vi "Periodic Tasks.vi"(11 "error in (no error)":errorcluster) -> ()   [LabVIEW 2012]
doc: "This VI runs in parallel to other tasks. It can contain as many user-defined periodic loops as you need. These can carry out PID or other sorts of timed response."
uses:
  <vilib>/Rock Robotics/WPI/DriverStation/DriverStationLCD/WPI_DriverStationLCDLCDLine.ctl
  <vilib>/Rock Robotics/SystemInterfaces/Utilities/FPGA_UtilitiesLED Source.ctl
  <vilib>/Rock Robotics/SystemInterfaces/Utilities/FPGA_UtilitiesLED State.ctl
  Robot Global Data.vi
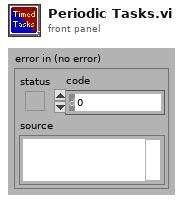
[diagram p1: front panel]
types:
  T1 = typedef "WPI_DriverStationLCDLCDLine.ctl" = enum16{"Main - Line 1", "User - Line 2", "User - Line 3", "User - Line 4", "User - Line 5", "User - Line 6"}
  T2 = cluster{"Case":dbl, "VisionTrack":bool, "ShootEnableWheels":bool, "Shoot":bool, "ManualExtend":dbl, "ManualRotate":dbl, "YCoord":dbl, "FlipUp":bool, "RotDeadband":dbl, "ExtDeadband":dbl, "ExtPOT":dbl, "RotPOT":dbl, "WheelFSpd":dbl, "WheelBSpd":dbl, "ServoPositions":cluster{"FlipperLeftUp":dbl, "FlipperLeftDown":dbl, "FlipperRightUp":dbl, "FlipperRightDown":dbl, "KickerLeftBack":dbl, "KickerLeftForward":dbl, "KickerRightBack":dbl, "KickerRightForward":dbl}, "POTPositions":cluster{"Setpoint 1":dbl, "Setpoint 2":dbl, "Setpoint 3":dbl, "Setpoint 4":dbl, "RotLow":dbl, "RotHigh":dbl, "ExtLow":dbl, "ExtHigh":dbl}, "ClimberHooked":bool}
  T3 = typedef "WPI_DigitalInputDevRef.ctl" = cluster{"DevStatus":errorcluster, "DIO Channel":T4, "Digital Module":T5}
  T4 = typedef "FPGA_DIOChannel.ctl" = enum8{"DIO 1", "DIO 2", "DIO 3", "DIO 4", "DIO 5", "DIO 6", "DIO 7", "DIO 8", "DIO 9", "DIO 10", "DIO 11", "DIO 12", "DIO 13", "DIO 14", "Invalid"}
  T5 = typedef "FPGA_TypedefDigitalModule.ctl" = enum16{"Digital Module 1", "Digital Module 2"}
  T6 = typedef "WPI_AnalogChannelDevRef.ctl" = cluster{"DevStatus":errorcluster, "Analog Module":T7, "Analog Channel":T8}
  T7 = typedef "FPGA_TypedefAnalogModule.ctl" = enum16{"Analog Module 1", "Analog Module 2"}
  T8 = typedef "FPGA_AIChannel.ctl" = enum8{"AI 1", "AI 2", "AI 3", "AI 4", "AI 5", "AI 6", "AI 7", "AI 8", "Invalid"}
  T9 = cluster{"FlipperLeftUp":dbl, "FlipperLeftDown":dbl, "FlipperRightUp":dbl, "FlipperRightDown":dbl, "KickerLeftBack":dbl, "KickerLeftForward":dbl, "KickerRightBack":dbl, "KickerRightForward":dbl}
  T10 = cluster{"Setpoint 1":dbl, "Setpoint 2":dbl, "Setpoint 3":dbl, "Setpoint 4":dbl, "RotLow":dbl, "RotHigh":dbl, "ExtLow":dbl, "ExtHigh":dbl}
  T11 = typedef "WPI_GyroDevRef.ctl" = cluster{"DevStatus":errorcluster, "Analog Module":T7, "Analog Channel":T8, "Offset":dbl, "Gain (VoltsPerDegree/Second)":dbl}
  T12 = typedef "WPI_EncoderDevRef.ctl" = cluster{"DevStatus":errorcluster, "EncoderIndex":T13, "CounterIndex":T14, "DistancePerCount":dbl, "Decoding Type":T15}
  T13 = typedef "FPGA_EncoderIdx.ctl" = enum8{"Enc 0", "Enc 1", "Enc 2", "Enc 3", "Invalid"}
  T14 = typedef "FPGA_CounterCtrSystemIndex.ctl" = enum8{"Ctr 0", "Ctr 1", "Ctr 2", "Ctr 3", "Ctr 4", "Ctr 5", "Ctr 6", "Ctr 7", "Invalid"}
  T15 = typedef "WPI_EncoderType.ctl" = enum16{"1x", "2x", "4x"}
  T16 = typedef "WPI_RelayValue.ctl" = enum16{"Off", "On", "Forward", "Reverse"}
  T17 = cluster{"Case":dbl, "Extension":dbl, "Rotation":dbl, "WheelF":dbl, "WheelB":dbl, "Left Kicker":dbl, "Right Kicker":dbl, "Left Flipper":dbl, "Right Flipper":dbl, "Lights":T16}
  T18 = typedef "FPGA_UtilitiesLED State.ctl" = enum16{"Off", "On", "Toggle"}
  T19 = typedef "FPGA_UtilitiesLED Source.ctl" = enum16{"User LED", "FPGA LED"}
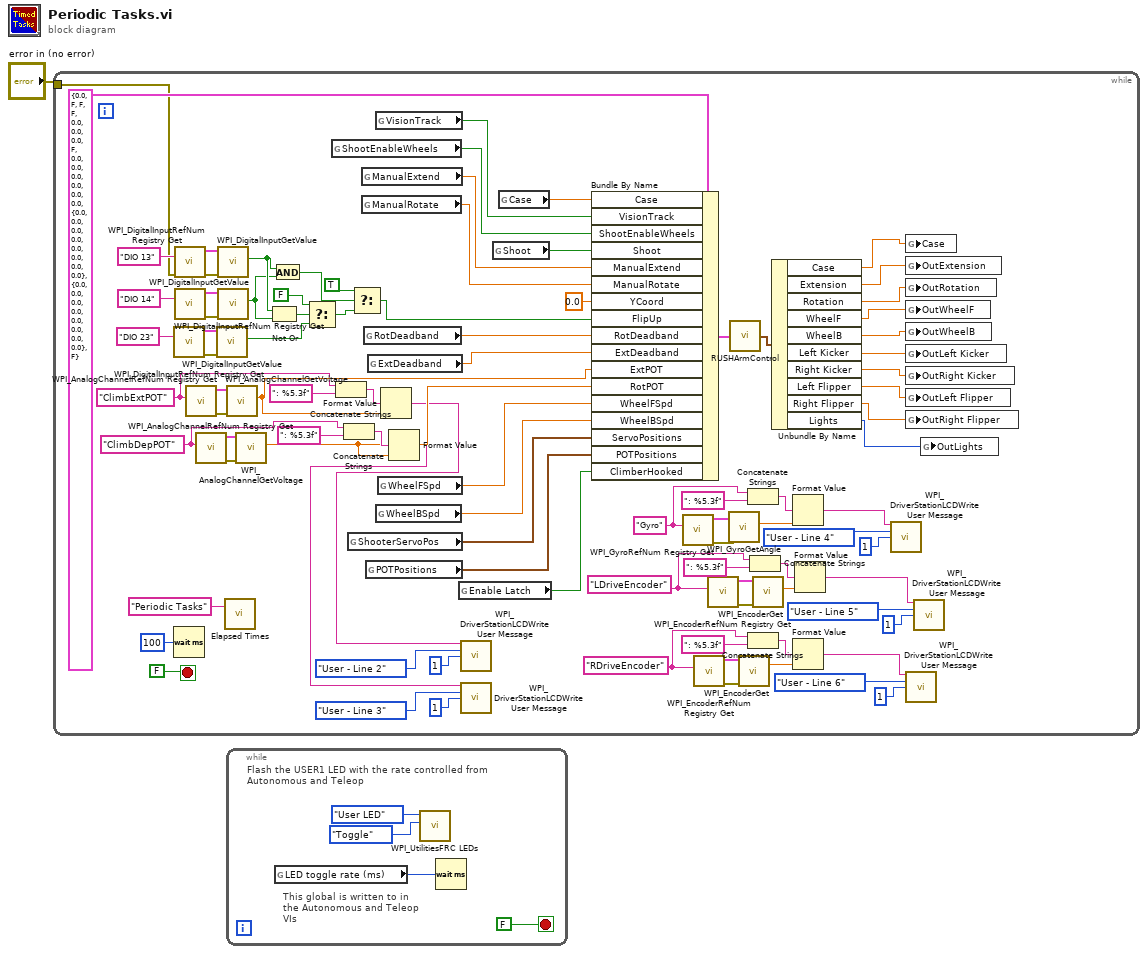
[diagram p0: block diagram]
diagram:
  n1 = while {
    tunnel: "error in (no error)" -> [w38]
    stop <- FALSE stop-if-true
    w8 = "ClimbExtPOT" ("refnum name")
    w19 = "RDriveEncoder" ("refnum name")
    w13 = "LDriveEncoder" ("refnum name")
    w4 = "ClimbDepPOT" ("refnum name")
    w31 = "Gyro" ("refnum name")
    n2 = call <vilib>:"WPI_DigitalInputRefNum Registry Get.vi"("refnum name"="DIO 23") -> ("error out"=w44:errorcluster, "DigitalInputDevRef"=w41:T3)  [unwired: 9 in]
    n3 = Wait (ms)(milliseconds to wait=u32 100) -> ()  [unwired: 1 out]
    n4 = call <vilib>:"WPI_DigitalInputRefNum Registry Get.vi"("error in (no error)"=w38, "refnum name"="DIO 13") -> ("error out"=w58:errorcluster, "DigitalInputDevRef"=w57:T3)  [unwired: 8 in]
    n5 = call <vilib>:"WPI_DigitalInputRefNum Registry Get.vi"("refnum name"="DIO 14") -> ("error out"=w53:errorcluster, "DigitalInputDevRef"=w54:T3)  [unwired: 9 in]
    n6 = call <vilib>:"WPI_AnalogChannelRefNum Registry Get.vi"("refnum name"=w8) -> ("error out"=w90:errorcluster, "AIDeviceRef"=w39:T6)  [unwired: 9 in]
    n7 = call <vilib>:"WPI_AnalogChannelRefNum Registry Get.vi"("refnum name"=w4) -> ("error out"=w85:errorcluster, "AIDeviceRef"=w84:T6)  [unwired: 9 in]
    n8 = call <vilib>:"WPI_DigitalInputGetValue.vi"("error in (no error)"=w44, "DigitalInputDevRef"=w41) -> ("Value"=w42:bool)  [unwired: 7 in, 2 out]
    n9 = call <vilib>:"WPI_DigitalInputGetValue.vi"("error in (no error)"=w58, "DigitalInputDevRef"=w57) -> ("Value"=w50:bool)  [unwired: 7 in, 2 out]
    n10 = call <vilib>:"WPI_DigitalInputGetValue.vi"("error in (no error)"=w53, "DigitalInputDevRef"=w54) -> ("Value"=w49:bool)  [unwired: 7 in, 2 out]
    n11 = call "Elapsed Times.vi"("Call Name"="Periodic Tasks") -> ()  [unwired: 2 in, 1 out]
    n12 = call <vilib>:"WPI_AnalogChannelGetVoltage.vi"("error in (no error)"=w90, "AIDeviceRef"=w39) -> ("Voltage"=w9:dbl)  [unwired: 7 in, 2 out]
    n13 = call <vilib>:"WPI_AnalogChannelGetVoltage.vi"("error in (no error)"=w85, "AIDeviceRef"=w84) -> ("Voltage"=w5:dbl)  [unwired: 7 in, 2 out]
    n14 = Not Or(1:w49, 2:w50) -> (0:w48:bool)
    n15 = And(x=w50, y=w49) -> (x .and. y?=w52:bool)
    n16 = Select(t=FALSE, s=w48, f=w42) -> (s? t:f=w46:bool)
    n17 = global read "Robot Global Data.vi" "ShootEnableWheels"() -> (w78:bool)
    n18 = Concatenate Strings(w8, ": %5.3f") -> (w10:string)
    n19 = Concatenate Strings(w4, ": %5.3f") -> (w7:string)
    n20 = global read "Robot Global Data.vi" "ShooterServoPos"() -> (w70:T9)
    n21 = Select(t=TRUE, s=w52, f=w46) -> (s? t:f=w45:bool)
    n22 = global read "Robot Global Data.vi" "ManualExtend"() -> (w76:dbl)
    n23 = global read "Robot Global Data.vi" "ManualRotate"() -> (w75:dbl)
    n24 = global read "Robot Global Data.vi" "RotDeadband"() -> (w74:dbl)
    n25 = global read "Robot Global Data.vi" "POTPositions"() -> (w69:T10)
    n26 = global read "Robot Global Data.vi" "ExtDeadband"() -> (w73:dbl)
    n27 = global read "Robot Global Data.vi" "VisionTrack"() -> (w79:bool)
    n28 = global read "Robot Global Data.vi" "WheelBSpd"() -> (w71:dbl)
    n29 = global read "Robot Global Data.vi" "WheelFSpd"() -> (w72:dbl)
    n30 = Format Value(format string=w10, value (0)=w9) -> (output string=w3:string)  [unwired: 1 in]
    n31 = Format Value(format string=w7, value (0)=w5) -> (output string=w2:string)  [unwired: 1 in]
    n32 = global read "Robot Global Data.vi" "Enable Latch"() -> (w40:bool)
    n33 = call <vilib>:"WPI_DriverStationLCDWrite User Message.vi"("line text"=w3, "line"=WPI_DriverStationLCDLCDLine."User - Line 2", "starting column"=i8 1) -> ()  [unwired: 2 in, 11 out]
    n34 = call <vilib>:"WPI_DriverStationLCDWrite User Message.vi"("line text"=w2, "line"=WPI_DriverStationLCDLCDLine."User - Line 3", "starting column"=i8 1) -> ()  [unwired: 2 in, 11 out]
    n35 = global read "Robot Global Data.vi" "Shoot"() -> (w77:bool)
    n36 = global read "Robot Global Data.vi" "Case"() -> (w80:dbl)
    n37 = Bundle By Name(cluster=T2 {"Case"=0.0, "VisionTrack"=FALSE, "ShootEnableWheels"=FALSE, "Shoot"=FALSE, "ManualExtend"=0.0, "ManualRotate"=0.0, "YCoord"=0.0, "FlipUp"=FALSE, "RotDeadband"=0.0, "ExtDeadband"=0.0, "ExtPOT"=0.0, "RotPOT"=0.0, "WheelFSpd"=0.0, "WheelBSpd"=0.0, "ServoPositions"={"FlipperLeftUp"=0.0, "FlipperLeftDown"=0.0, "FlipperRightUp"=0.0, "FlipperRightDown"=0.0, "KickerLeftBack"=0.0, "KickerLeftForward"=0.0, "KickerRightBack"=0.0, "KickerRightForward"=0.0}, "POTPositions"={"Setpoint 1"=0.0, "Setpoint 2"=0.0, "Setpoint 3"=0.0, "Setpoint 4"=0.0, "RotLow"=0.0, "RotHigh"=0.0, "ExtLow"=0.0, "ExtHigh"=0.0}, "ClimberHooked"=FALSE} ("In Cluster"), "Case"=w80, "VisionTrack"=w79, "ShootEnableWheels"=w78, "Shoot"=w77, "ManualExtend"=w76, "ManualRotate"=w75, "YCoord"=0.0, "FlipUp"=w45, "RotDeadband"=w74, "ExtDeadband"=w73, "ExtPOT"=w9, "RotPOT"=w5, "WheelFSpd"=w72, "WheelBSpd"=w71, "ServoPositions"=w70, "POTPositions"=w69, "ClimberHooked"=w40) -> (w82:T2)
    n38 = call <vilib>:"WPI_GyroRefNum Registry Get.vi"("refnum name"=w31) -> ("error out"=w91:errorcluster, "GyroDevRef"=w92:T11)  [unwired: 9 in]
    n39 = call <vilib>:"WPI_EncoderRefNum Registry Get.vi"("refnum name"=w19) -> ("error out"=w87:errorcluster, "EncoderDevRef"=w86:T12)  [unwired: 9 in]
    n40 = call <vilib>:"WPI_EncoderRefNum Registry Get.vi"("refnum name"=w13) -> ("error out"=w88:errorcluster, "EncoderDevRef"=w89:T12)  [unwired: 9 in]
    n41 = call <vilib>:"WPI_GyroGetAngle.vi"("error in (no error)"=w91, "GyroDevRef"=w92) -> ("Angle"=w24:dbl)  [unwired: 6 in, 3 out]
    n42 = call "RUSHArmControl.vi"("In Cluster"=w82) -> ("Out Cluster"=w81:T17)
    n43 = call <vilib>:"WPI_EncoderGet.vi"("error in (no error)"=w87, "EncoderDevRef"=w86) -> ("Distance"=w18:dbl)  [unwired: 4 in, 5 out]
    n44 = Concatenate Strings(w31, ": %5.3f") -> (w22:string)
    n45 = Concatenate Strings(w19, ": %5.3f") -> (w20:string)
    n46 = Concatenate Strings(w13, ": %5.3f") -> (w15:string)
    n47 = call <vilib>:"WPI_EncoderGet.vi"("error in (no error)"=w88, "EncoderDevRef"=w89) -> ("Distance"=w14:dbl)  [unwired: 4 in, 5 out]
    n48 = Unbundle By Name(w81) -> ("Case"=w68:dbl, "Extension"=w67:dbl, "Rotation"=w66:dbl, "WheelF"=w65:dbl, "WheelB"=w64:dbl, "Left Kicker"=w63:dbl, "Right Kicker"=w62:dbl, "Left Flipper"=w61:dbl, "Right Flipper"=w60:dbl, "Lights"=w59:T16)
    n49 = Format Value(format string=w22, value (0)=w24) -> (output string=w23:string)  [unwired: 1 in]
    n50 = Format Value(format string=w20, value (0)=w18) -> (output string=w17:string)  [unwired: 1 in]
    n51 = Format Value(format string=w15, value (0)=w14) -> (output string=w12:string)  [unwired: 1 in]
    n52 = call <vilib>:"WPI_DriverStationLCDWrite User Message.vi"("line text"=w23, "line"=WPI_DriverStationLCDLCDLine."User - Line 4", "starting column"=i8 1) -> ()  [unwired: 2 in, 11 out]
    n53 = global write "Robot Global Data.vi" "Case"(w68) -> ()
    n54 = global write "Robot Global Data.vi" "OutExtension"(w67) -> ()
    n55 = global write "Robot Global Data.vi" "OutRotation"(w66) -> ()
    n56 = global write "Robot Global Data.vi" "OutWheelF"(w65) -> ()
    n57 = global write "Robot Global Data.vi" "OutWheelB"(w64) -> ()
    n58 = global write "Robot Global Data.vi" "OutLeft Kicker"(w63) -> ()
    n59 = global write "Robot Global Data.vi" "OutRight Kicker"(w62) -> ()
    n60 = global write "Robot Global Data.vi" "OutLeft Flipper"(w61) -> ()
    n61 = global write "Robot Global Data.vi" "OutRight Flipper"(w60) -> ()
    n62 = call <vilib>:"WPI_DriverStationLCDWrite User Message.vi"("line text"=w17, "line"=WPI_DriverStationLCDLCDLine."User - Line 6", "starting column"=i8 1) -> ()  [unwired: 2 in, 11 out]
    n63 = call <vilib>:"WPI_DriverStationLCDWrite User Message.vi"("line text"=w12, "line"=WPI_DriverStationLCDLCDLine."User - Line 5", "starting column"=i8 1) -> ()  [unwired: 2 in, 11 out]
    n64 = global write "Robot Global Data.vi" "OutLights"(w59) -> ()
  }
  n65 = while {
    stop <- FALSE stop-if-true
    # "This global is written to in the Autonomous and Teleop VIs"
    # "Flash the USER1 LED with the rate controlled from Autonomous and Teleop"
    n66 = global read "Robot Global Data.vi" "LED toggle rate (ms)"() -> (w96:u32)
    n67 = call <vilib>:"WPI_UtilitiesFRC LEDs.vi"("State"=FPGA_UtilitiesLED_State."Toggle", "LED Type"=FPGA_UtilitiesLED_Source."User LED") -> ()  [unwired: 1 in, 9 out]
    n68 = Wait (ms)(milliseconds to wait=w96) -> ()  [unwired: 1 out]
  }
